vi "test Loopback.vi"(8 "error in":errorcluster, 11 "TestCase in":refnum<class "Single Core Simple Loopback.lvclass">) -> (0 "error out":errorcluster, 3 "TestCase out":refnum<class "Single Core Simple Loopback.lvclass">)   [LabVIEW 2020, in "Single Core Simple Loopback.lvclass"]
uses:
  Single Core Simple Loopback.lvclass
  C:/Program Files (x86)/National Instruments/LabVIEW 2020/vi.lib/addons/_JKI Toolkits/VI Tester/TestCase.llb/TestCase.lvclass
  <vilib>/addons/_JKI Toolkits/VI Tester/TestCase.llb/TestCase.lvclass
  niveristand-custom-device-testing-tools/VeriStandTestUtilities/VeriStandTestUtilities.lvlib
  <vilib>/numeric/Random Number (Range) I64.vi
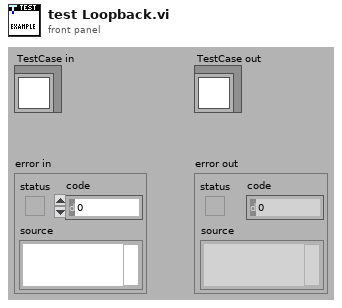
[diagram p1: front panel]
types:
  T1 = typedef "NI_VS Workspace ExecutionAPI.lvlib/WorkspaceAPI.ctl" = refnum<k24>
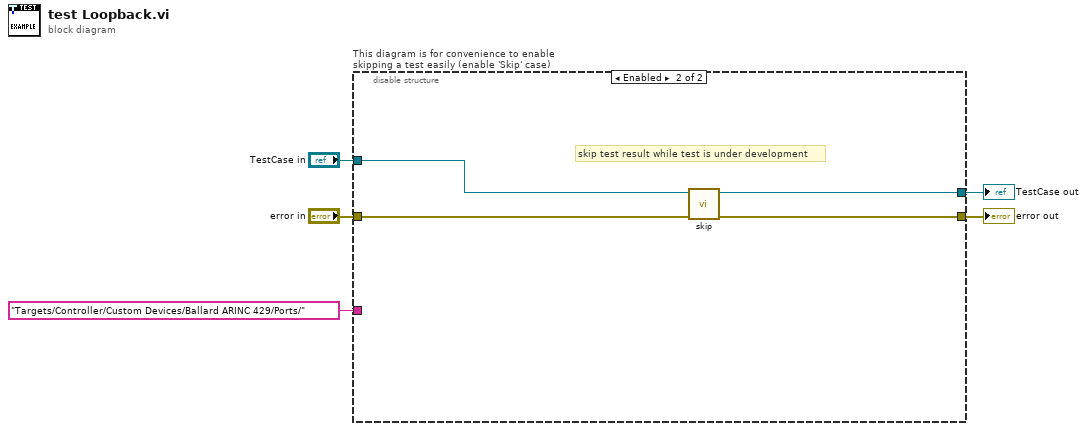
[diagram p0: block diagram]
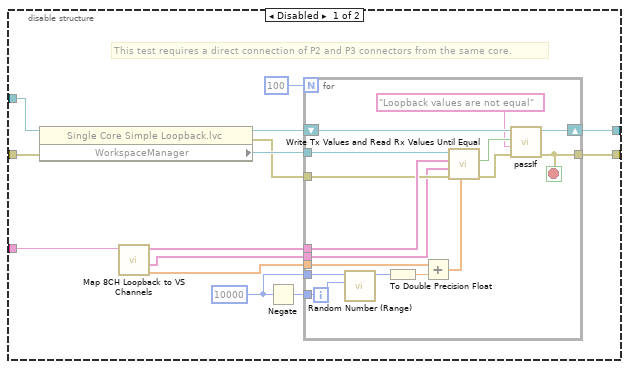
[diagram p2: hidden frame]
diagram:
  n1 = disable-structure "This diagram is for convenience to enable skipping a test easily (enable 'Skip' case)" shown="Enabled" {
    disable-tunnel: "TestCase in" -> [w9 w39]
    disable-tunnel: [w7 w37] -> w2
    disable-tunnel: [w6 w38] -> w4
    disable-tunnel: "error in" -> [w8 w36]
    disable-tunnel: "Targets/Controller/Custom Devices/Ballard ARINC 429/Ports/" ("Channel") -> [w12 _]
    frame Disabled {
      w19 = i64 10000 ("upper bound (100)")
      # "This test requires a direct connection of P2 and P3 connectors from the same core."
      n2 = property class="Single Core Simple Loopback.lvc"(reference=w9, error in=w8) -> (reference out=w14:refnum<class "Single Core Simple Loopback.lvclass">, error out=w15:errorcluster, "WorkspaceManager"=w16:T1)
      n3 = call "Map 8CH Loopback to VS Channels.vi"("Base Path to Ports"=w12) -> ("Channel Count"=w10:dbl[], "Rx Channel Array"=w11:string[], "Tx Channel Array"=w17:string[])  [unwired: 7 in, 1 out]
      n4 = Negate(x=w19) -> (-x=w18:i64)
      n5 = for {
        N: 100 -> [_]
        tunnel: w10 -> [w33]
        tunnel: w19 -> [w32]
        tunnel: w18 -> [w31]
        tunnel: w17 -> [w30]
        tunnel: w16 -> [w29]
        tunnel: w15 -> [w28]
        tunnel: w11 -> [w27]
        shift-right: [w24] -> w7
        shift-left: w14 -> [w25]
        tunnel: [w22] -> w6
        stop <- w22 stop-if-true
        n6 = call-poly <vilib>:"Random Number (Range).vi"("lower bound (-100)"=w31, "upper bound (100)"=w32) -> ("number"=w35:i64)  [unwired: 9 in]
        n7 = To Double Precision Float(number=w35) -> (double precision float=w34:dbl)
        n8 = Add(x=w33, y=w34) -> (x+y=w23:dbl[])
        n9 = call "Write Tx Values and Read Rx Values Until Equal.vi"("Tx values"=w23, "error in"=w28, "Rx aliases"=w27, "Tx aliases"=w30, "workspace manager in"=w29) -> ("error out"=w26:errorcluster, "values equal"=w21:bool)  [unwired: 4 in, 1 out]
        n10 = call-dynamic "passIf.vi"("error in (no error)"=w26, "message (\"\")"="Loopback values are not equal" ("message (\"\")"), "pass"=w21, "TestCase in"=w25) -> ("error out"=w22:errorcluster, "TestCase out"=w24:refnum<class "Single Core Simple Loopback.lvclass">)  [unwired: 6 in]
      }
    }
    frame Enabled {
      # "skip test result while test is under development"
      n11 = call <vilib>:"skip.vi"("error in (no error)"=w36, "TestCase in"=w39) -> ("error out"=w38:errorcluster, "TestCase out"=w37:refnum<class "Single Core Simple Loopback.lvclass">)  [unwired: 8 in]
    }
  }
  "error out" <- w4
  "TestCase out" <- w2
